vi "Disable Source Separation.vi"(8 "Error In":errorcluster, 9 "Operation Start Time":timestamp, 11 "Root Path":path) -> (0 "Error Out":errorcluster)   [LabVIEW 2014]
doc: "Copyright (c) 2018 Sze Howe Koh\n\nThis Source Code Form is subject to the terms of the Mozilla Public License, v. 2.0. If a copy of the MPL was not distributed with this file, You can obtain one at http://mozilla.org/MPL/2.0/."
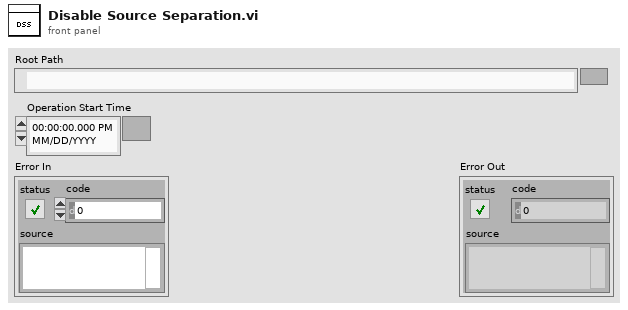
[diagram p1: front panel]
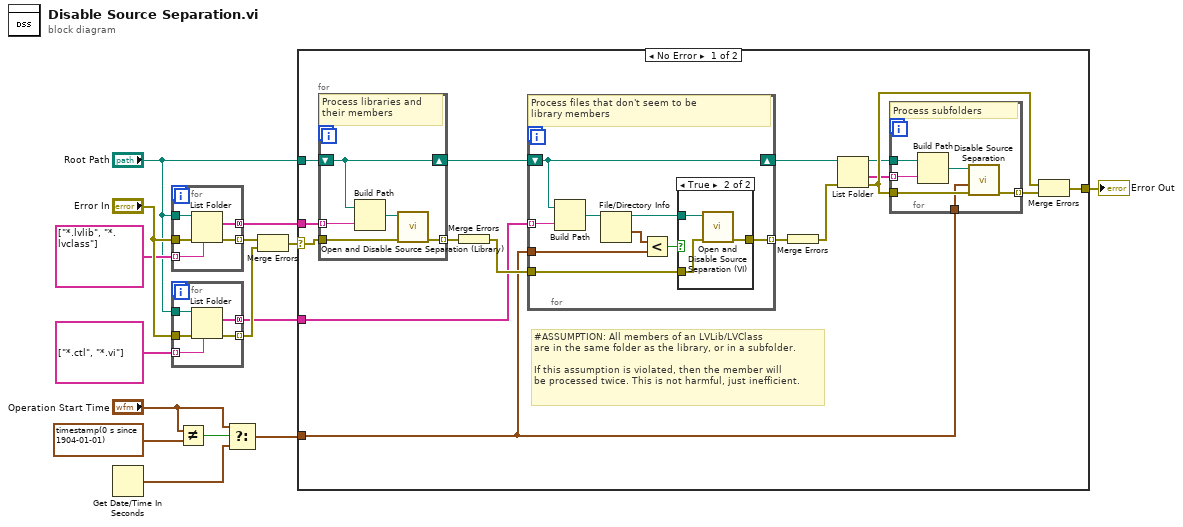
[diagram p0: block diagram]
diagram:
  n1 = Get Date/Time In Seconds() -> (seconds since 1Jan1904=w5:timestamp)
  n2 = for {
    tunnel: "Root Path" -> [w20]
    tunnel: [w19] -> w12 mode=concatenating
    tunnel: string[] ["*.lvlib", "*.lvclass"] -> [w18] mode=indexing
    tunnel: "Error In" -> [w17]
    tunnel: [w16] -> w3 mode=indexing
    n3 = List Folder(path=w20, pattern=w18, error in=w17) -> (filenames=w19:string[], error out=w16:errorcluster)  [unwired: 1 in, 2 out]
  }
  n4 = for {
    tunnel: "Root Path" -> [w25]
    tunnel: [w24] -> w9 mode=concatenating
    tunnel: string[] ["*.ctl", "*.vi"] -> [w23] mode=indexing
    tunnel: "Error In" -> [w22]
    tunnel: [w21] -> w15 mode=indexing
    n5 = List Folder(path=w25, pattern=w23, error in=w22) -> (filenames=w24:string[], error out=w21:errorcluster)  [unwired: 1 in, 2 out]
  }
  n6 = Not Equal?(x="Operation Start Time", y=timestamp(0 s since 1904-01-01)) -> (x != y?=w7:bool)
  n7 = Select(t="Operation Start Time", s=w7, f=w5) -> (s? t:f=w4:timestamp)
  n8 = Merge Errors(w3, w15) -> (w1:errorcluster)
  n9 = case shown="No Error" w1 {
    selector: w1 -> [w26 w66]
    tunnel: w12 -> [w39 _]
    tunnel: "Root Path" -> [w38 _]
    tunnel: w9 -> [w37 _]
    tunnel: w4 -> [w32 _]
    tunnel: [w27 w66] -> w2
    frame No Error {
      # "#ASSUMPTION: All members of an LVLib/LVClass\nare in the same folder as the library, or in a subfolder.\n\nIf this assumption is violated, then the member will\nbe processed twice. This is not harmful, just inefficient."
      n10 = for {
        tunnel: w39 -> [w59] mode=indexing
        shift-right: [w57] -> w34
        shift-left: w38 -> [w57]
        tunnel: w26 -> [w56]
        tunnel: [w55] -> w31 mode=indexing
        # "Process libraries and\ntheir members"
        n11 = Build Path(base path=w57, name or relative path=w59) -> (appended path=w58:path)
        n12 = call "Open and Disable Source Separation (Library).vi"("Error In"=w56, "Library Path"=w58) -> ("Error Out"=w55:errorcluster)  [unwired: 9 in]
      }
      n13 = Merge Errors(w31) -> (w40:errorcluster)
      n14 = for {
        tunnel: w37 -> [w50] mode=indexing
        tunnel: w32 -> [w49]
        shift-right: [w44] -> w33
        shift-left: w34 -> [w44]
        tunnel: w40 -> [w43]
        tunnel: [w42] -> w30 mode=indexing
        # "Process files that don't seem to be\nlibrary members"
        n15 = Build Path(base path=w44, name or relative path=w50) -> (appended path=w48:path)
        n16 = File/Directory Info(path=w48) -> (path out=w45:path, last mod=w47:timestamp)  [unwired: 1 in, 5 out]
        n17 = Less?(x=w47, y=w49) -> (x < y?=w46:bool)
        n18 = case shown="True" w46 {
          tunnel: w45 -> [_ w54]
          tunnel: w43 -> [w51 w53]
          tunnel: [w51 w52] -> w42
          frame False {
          }
          frame True {
            n19 = call "Open and Disable Source Separation (VI).vi"("Error In"=w53, "VI Path"=w54) -> ("Error Out"=w52:errorcluster)  [unwired: 9 in]
          }
        }
      }
      n20 = Merge Errors(w30) -> (w29:errorcluster)
      n21 = List Folder(path=w33, error in=w29) -> (path out=w36:path, folder names=w35:string[], error out=w41:errorcluster)  [unwired: 2 in, 1 out]
      n22 = for {
        tunnel: w36 -> [w64]
        tunnel: w35 -> [w63] mode=indexing
        tunnel: w32 -> [w61]
        tunnel: w41 -> [w65]
        tunnel: [w60] -> w28 mode=indexing
        # "Process subfolders"
        n23 = Build Path(base path=w64, name or relative path=w63) -> (appended path=w62:path)
        n24 = call "Disable Source Separation.vi"("Error In"=w65, "Operation Start Time"=w61, "Root Path"=w62) -> ("Error Out"=w60:errorcluster)  [unwired: 8 in]
      }
      n25 = Merge Errors(w41, w28) -> (w27:errorcluster)
    }
    frame Error {
    }
  }
  "Error Out" <- w2
